vi "Set Variable Value.vi"(8 "error in (no error)":errorcluster, 9 "varValue":dbl, 10 "varName":string, 11 "muExpr in":refnum<class "muExpr.lvclass">) -> (0 "error out":errorcluster, 3 "muExpr out":refnum<class "muExpr.lvclass">)   [LabVIEW 2015, in "muParser.lvlib" / "muExpr.lvclass"]
uses:
  muExpr.lvclass
  muExpr.lvclass/muExpr.ctl
  muParser.lvlib
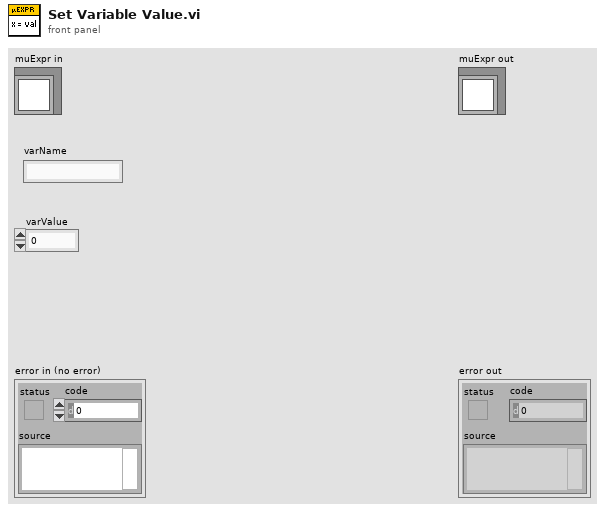
[diagram p1: front panel]
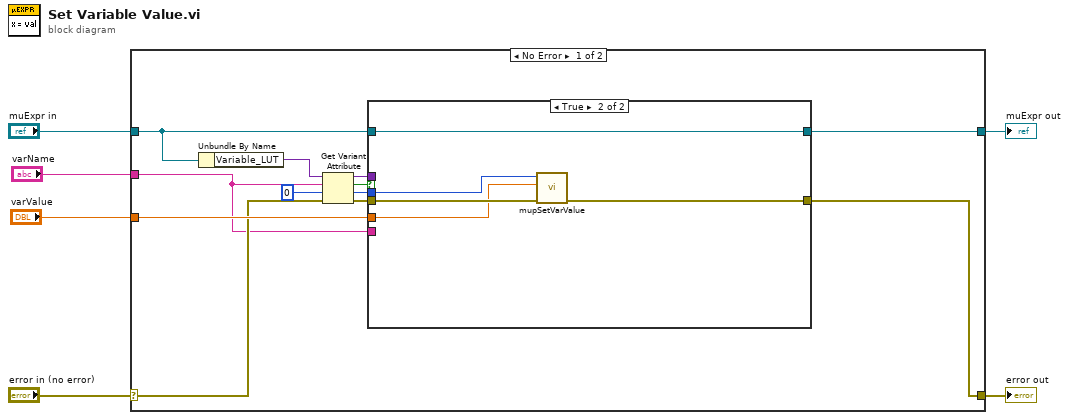
[diagram p0: block diagram]
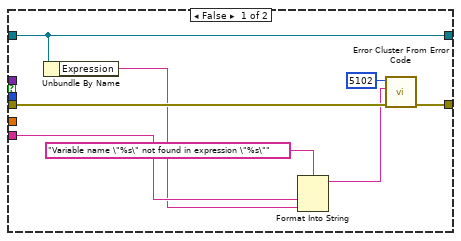
[diagram p2: hidden frame]
diagram:
  n1 = case shown="No Error" "error in (no error)" {
    selector: "error in (no error)" -> [w13 w33]
    tunnel: [w12 w33] -> w5
    tunnel: [w7 w32] -> w3
    tunnel: "muExpr in" -> [w9 w32]
    tunnel: "varValue" -> [w16 _]
    tunnel: "varName" -> [w10 _]
    frame No Error {
      n2 = Unbundle By Name(w9) -> ("Variable_LUT"=w18:variant)
      n3 = Get Variant Attribute(Variant=w18, name=w10, default value (empty Variant)=u64 0 ("pd"), error in=w13) -> (duplicate Variant=w8:variant, found=w11:bool, value=w14:u64, error out=w17:errorcluster)
      n4 = case shown="True" w11 {
        tunnel: w17 -> [w26 w30]
        tunnel: w16 -> [_ w28]
        tunnel: w14 -> [_ w27]
        tunnel: [w24 w29] -> w12
        tunnel: w10 -> [w23 _]
        tunnel: w9 -> [w25 w31]
        tunnel: w8 -> [_ _]
        tunnel: [w25 w31] -> w7
        frame False {
          n5 = Unbundle By Name(w25) -> ("Expression"=w20:string)
          n6 = Format Into String(format string="Variable name \"%s\" not found in expression \"%s\"", w23, w20) -> (resulting string=w19:string)  [unwired: 2 in, 1 out]
          n7 = call <vilib>:"Error Cluster From Error Code.vi"("error in (no error)"=w26, "error message (\"\")"=w19, "error code (0)"=5102) -> ("error out"=w24:errorcluster)  [unwired: 6 in]
        }
        frame True {
          n8 = call "mupSetVarValue.vi"("error in (no error)"=w30, "varValue"=w28, "varPtr in"=w27) -> ("error out"=w29:errorcluster)  [unwired: 7 in, 1 out]
        }
      }
    }
    frame Error {
    }
  }
  "error out" <- w5
  "muExpr out" <- w3
